vi "error tails.vi"(1 "Tails":dbl) -> (0 "Tails error":dbl)   [LabVIEW 2016]
doc: "This is the tails contribution to the internal error"
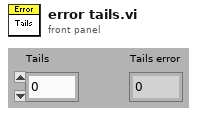
[diagram p1: front panel]
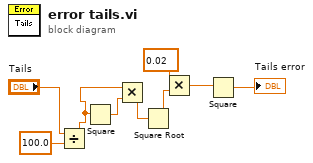
[diagram p0: block diagram]
diagram:
  n1 = Divide(x="Tails", y=100.0) -> (x/y=w1:dbl)
  n2 = Square(x=w1) -> (x^2=w4:dbl)
  n3 = Multiply(x=w1, y=w4) -> (x*y=w7:dbl)
  n4 = Square Root(x=w7) -> (sqrt(x)=w8:dbl)
  n5 = Multiply(x=0.02, y=w8) -> (x*y=w6:dbl)
  n6 = Square(x=w6) -> (x^2=→"Tails error":dbl)
